vi "appendXMLReverse.vi"(8 "Reverse":cluster{"Reverse X":bool, "Reverse Y":bool}, 9 "error in (no error)":errorcluster, 10 "Parent Camera Node":refnum<k20>, 11 "DOM document out":refnum<k20>) -> (0 "error out":errorcluster)   [LabVIEW 2013]
uses:
  <resource>/objmgr/DOMUserDefRef.rc
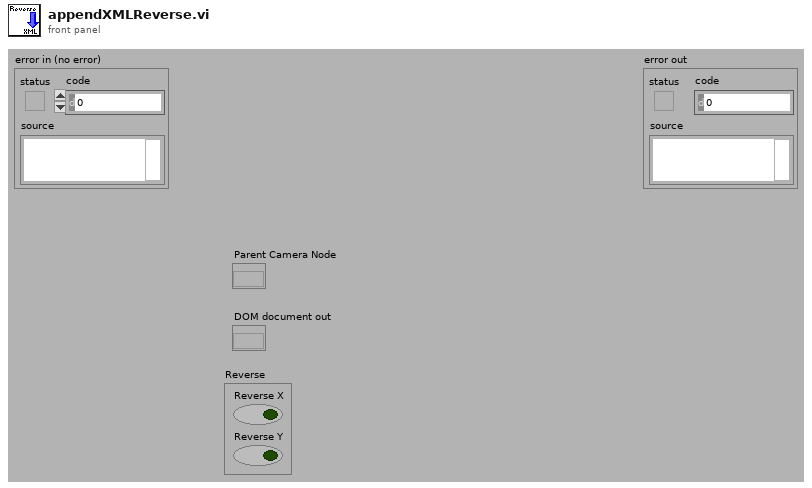
[diagram p1: front panel]
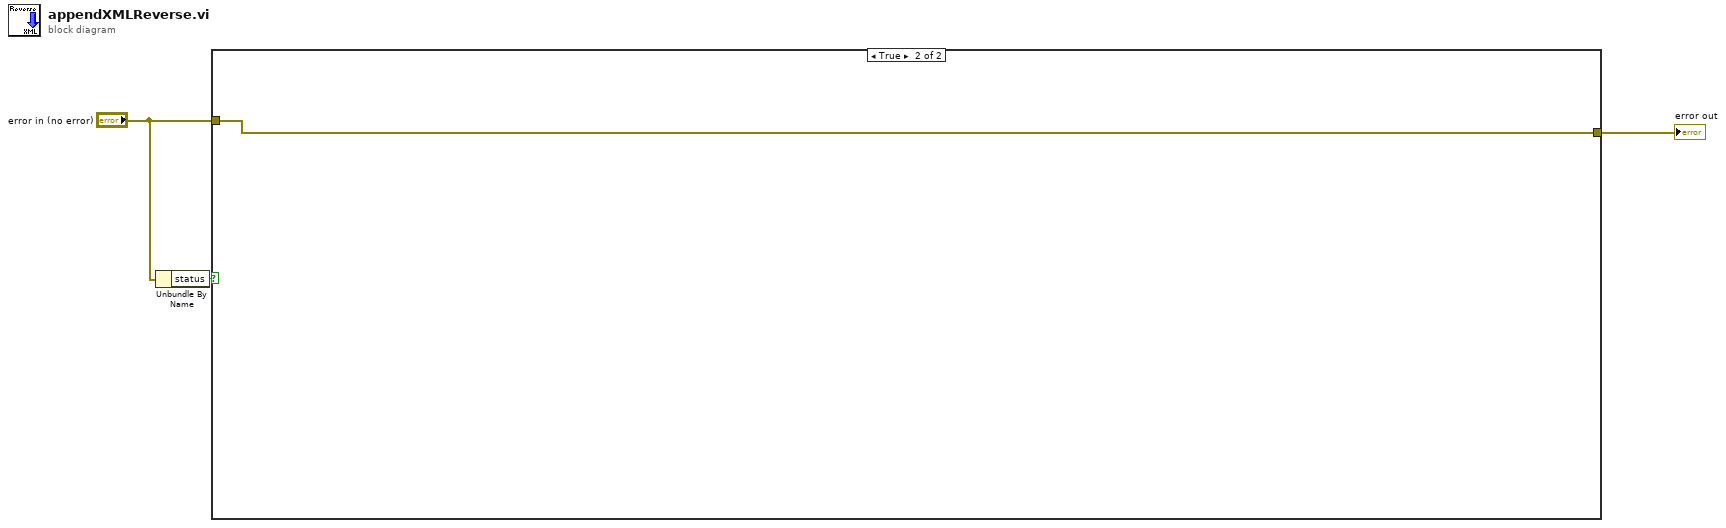
[diagram p0: block diagram]
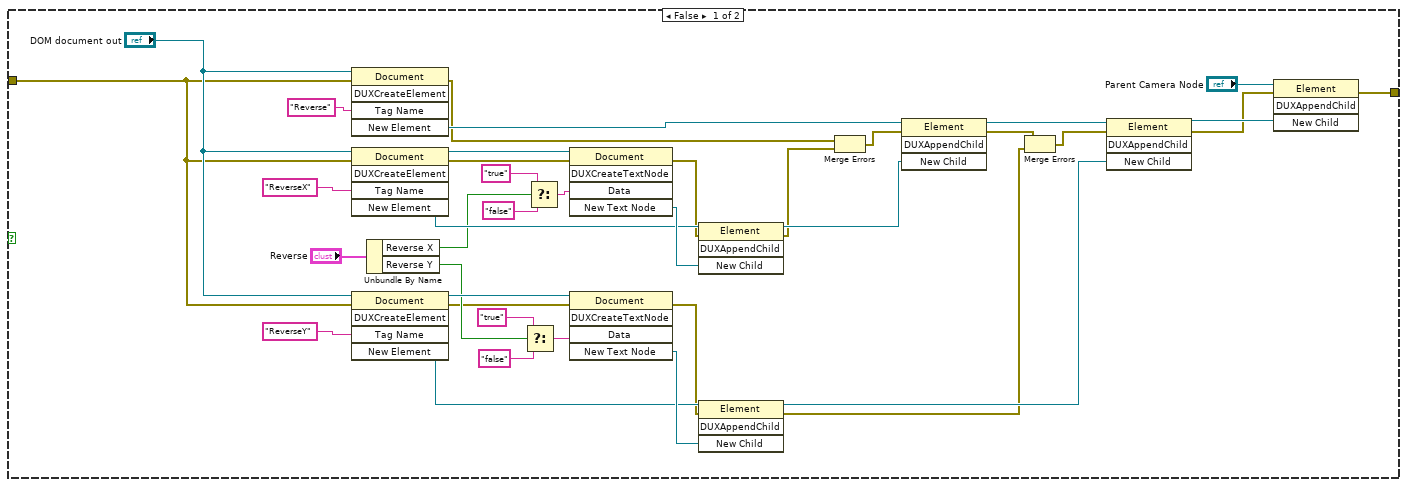
[diagram p2: hidden frame]
diagram:
  n1 = Unbundle By Name("error in (no error)") -> ("status"=w2:bool)
  n2 = case shown="True" w2 {
    tunnel: "error in (no error)" -> [w16 w42]
    tunnel: [w4 w42] -> w3
    frame False {
      n3 = invoke class="Document" method="DUXCreateElement"(reference="DOM document out", error in=w16, "Tag Name"="Reverse") -> (error out=w11:errorcluster, "New Element"=w36:refnum<k20>)  [unwired: 2 in, 3 out]
      n4 = invoke class="Document" method="DUXCreateElement"(reference="DOM document out", error in=w16, "Tag Name"="ReverseX") -> (reference out=w35:refnum<k20>, error out=w15:errorcluster, "New Element"=w31:refnum<k20>)  [unwired: 2 in, 2 out]
      n5 = invoke class="Document" method="DUXCreateElement"(reference="DOM document out", error in=w16, "Tag Name"="ReverseY") -> (reference out=w38:refnum<k20>, error out=w14:errorcluster, "New Element"=w33:refnum<k20>)  [unwired: 2 in, 2 out]
      n6 = Unbundle By Name("Reverse") -> ("Reverse X"=w26:bool, "Reverse Y"=w21:bool)
      n7 = Select(t="true" ("Tag Name"), s=w21, f="false" ("Tag Name")) -> (s? t:f=w23:string)
      n8 = Select(t="true" ("Tag Name"), s=w26, f="false" ("Tag Name")) -> (s? t:f=w22:string)
      n9 = invoke class="Document" method="DUXCreateTextNode"(reference=w35, error in=w15, "Data"=w22) -> (error out=w12:errorcluster, "New Text Node"=w32:refnum<k20>)  [unwired: 2 in, 3 out]
      n10 = invoke class="Document" method="DUXCreateTextNode"(reference=w38, error in=w14, "Data"=w23) -> (error out=w13:errorcluster, "New Text Node"=w34:refnum<k20>)  [unwired: 2 in, 3 out]
      n11 = invoke class="Element" method="DUXAppendChild"(reference=w31, error in=w12, "New Child"=w32) -> (reference out=w30:refnum<k20>, error out=w10:errorcluster)  [unwired: 1 in, 2 out]
      n12 = invoke class="Element" method="DUXAppendChild"(reference=w33, error in=w13, "New Child"=w34) -> (reference out=w29:refnum<k20>, error out=w6:errorcluster)  [unwired: 1 in, 2 out]
      n13 = Merge Errors(w11, w10) -> (w9:errorcluster)
      n14 = invoke class="Element" method="DUXAppendChild"(reference=w36, error in=w9, "New Child"=w30) -> (reference out=w37:refnum<k20>, error out=w8:errorcluster)  [unwired: 1 in, 2 out]
      n15 = Merge Errors(w8, w6) -> (w7:errorcluster)
      n16 = invoke class="Element" method="DUXAppendChild"(reference=w37, error in=w7, "New Child"=w29) -> (reference out=w17:refnum<k20>, error out=w5:errorcluster)  [unwired: 1 in, 2 out]
      n17 = invoke class="Element" method="DUXAppendChild"(reference="Parent Camera Node", error in=w5, "New Child"=w17) -> (error out=w4:errorcluster)  [unwired: 1 in, 3 out]
    }
    frame True {
    }
  }
  "error out" <- w3
